vi "LV Dev Doc - Instantiate with Ref.vi"(5 "VI Refnum":refnum<vi>, 11 "error in (no error)":errorcluster) -> (4 "Document.lvclass":refnum<class "Document.lvclass">, 15 "error out":errorcluster)   [LabVIEW 2016, in "LV DEV.lvclass"]
uses:
  LV DEV.lvclass
  Document.lvclass
  D:/MDI Project/source code/Document/Document.lvclass
  D:/MDI Project/source code/Document/Child Classes/LV Doc/LV Doc.lvclass
  LV Doc.lvclass/LV Doc.ctl
  LV Doc.lvclass
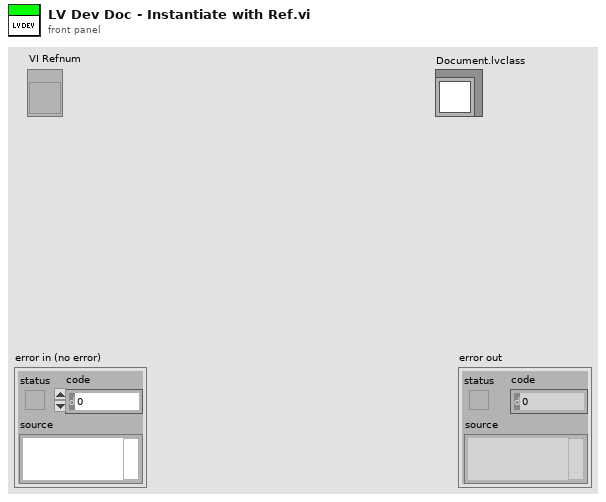
[diagram p1: front panel]
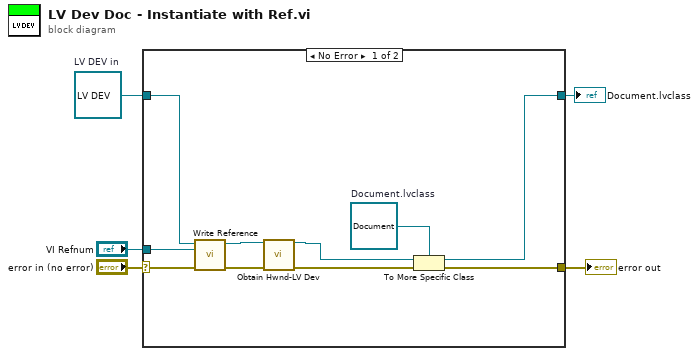
[diagram p0: block diagram]
diagram:
  w3 = refnum<class "LV DEV.lvclass"> refnum  # LV DEV in
  n1 = case shown="No Error" "error in (no error)" {
    selector: "error in (no error)" -> [w14 w17]
    tunnel: [w11 w17] -> w4
    tunnel: [w10 w16] -> w2
    tunnel: w3 -> [w13 w16]
    tunnel: "VI Refnum" -> [w12 _]
    frame No Error {
      w15 = refnum<class "Document.lvclass"> refnum  # Document.lvclass
      n2 = call "Write Reference.vi"("error in (no error)"=w14, "Reference"=w12, "LV Doc in"=w13) -> ("error out"=w7:errorcluster, "LV Doc out"=w9:refnum<class "LV DEV.lvclass">)  [unwired: 7 in]
      n3 = call-dynamic "Obtain Hwnd-LV Dev.vi"("LV DEV in"=w9, "error in (no error)"=w7) -> ("LV DEV out"=w8:refnum<class "LV DEV.lvclass">, "error out"=w6:errorcluster)  [unwired: 12 in]
      n4 = To More Specific Class(target class=w15, reference=w8, error in=w6) -> (specific class reference=w10:refnum<class "Document.lvclass">, error out=w11:errorcluster)
    }
    frame Error {
    }
  }
  "error out" <- w4
  "Document.lvclass" <- w2
